vi "BD CleanUp.vi"(8 "error in (no error)":errorcluster, 10 "Clean Up Options":T1, 11 "Block Diagram in":refnum<vi>) -> (0 "error out":errorcluster, 3 "Block Diagram out":refnum<vi>)   [LabVIEW 2019, in "gRPC Template Creation Utility.lvlib"]
uses:
  gRPC Template Creation Utility.lvlib
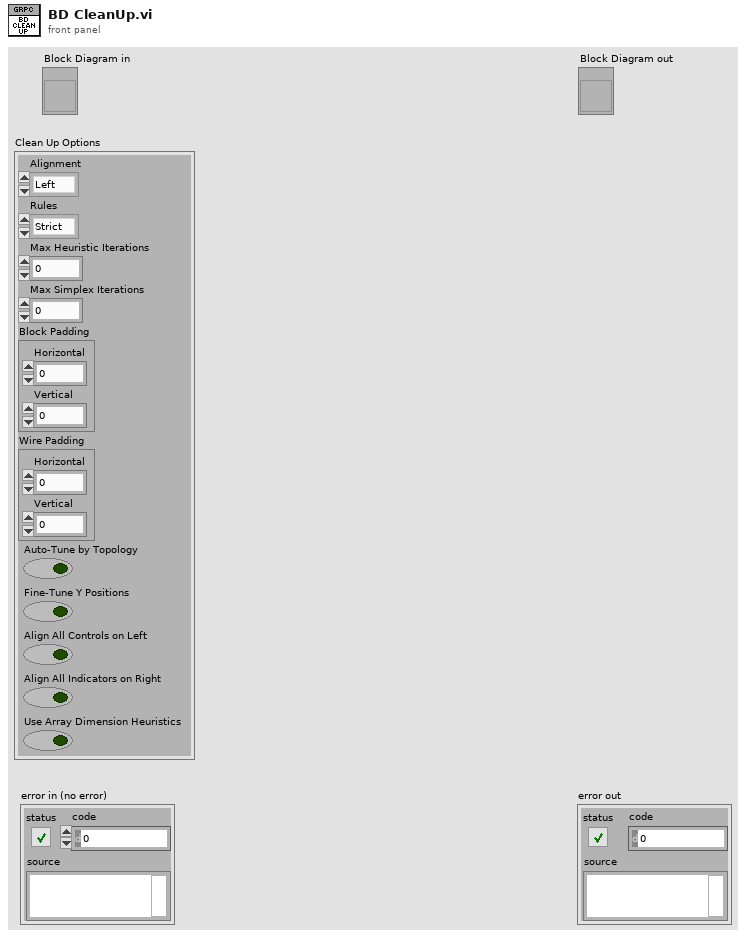
[diagram p1: front panel]
types:
  T1 = cluster{"Alignment":enum32{"Left", "Right", "Hybrid", "Center", "Gravity"}, "Rules":enum32{"Strict", "Allow Wires Under Labels", "Allow Wires Under Lead Nodes", "Allow Wires Under Wide Blocks"}, "Max Heuristic Iterations":u32, "Max Simplex Iterations":u32, "Block Padding":cluster{"Horizontal":i32, "Vertical":i32}, "Wire Padding":cluster{"Horizontal":i32, "Vertical":i32}, "Auto-Tune by Topology":bool, "Fine-Tune Y Positions":bool, "Align All Controls on Left":bool, "Align All Indicators on Right":bool, "Use Array Dimension Heuristics":bool}
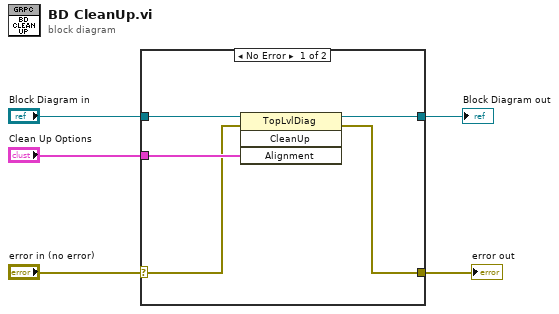
[diagram p0: block diagram]
diagram:
  n1 = case shown="No Error" "error in (no error)" {
    selector: "error in (no error)" -> [w6 w11]
    tunnel: "Block Diagram in" -> [w10 w12]
    tunnel: "Clean Up Options" -> [w9 _]
    tunnel: [w8 w12] -> w3
    tunnel: [w7 w11] -> w2
    frame No Error {
      n2 = invoke class="TopLvlDiag" method="CleanUp"(reference=w10, error in=w6, "Alignment"=w9) -> (reference out=w8:refnum<vi>, error out=w7:errorcluster)  [unwired: 1 in, 2 out]
    }
    frame Error {
    }
  }
  "Block Diagram out" <- w3
  "error out" <- w2
